vi "AlazarDSPSetParameterU32.vi"(4 "error in (no error)":errorcluster, 5 "value":u32, 6 "Parameter":u32(ring) items=["Raw+FFT supported", "FFT subtractor supported"], 7 "DSP Handle":u64) -> (0 "error out":errorcluster, 1 "Return Code":u32, 3 "DSP Handle":u64)   [LabVIEW 2009]
doc: "Get a device attribute as a signed long value."
uses:
  ATSApi.dll
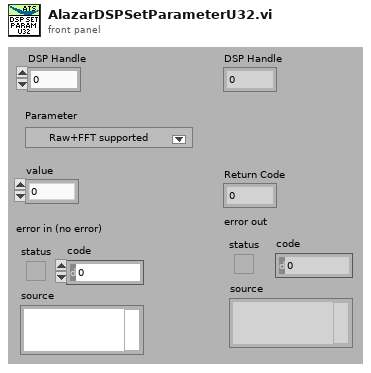
[diagram p1: front panel]
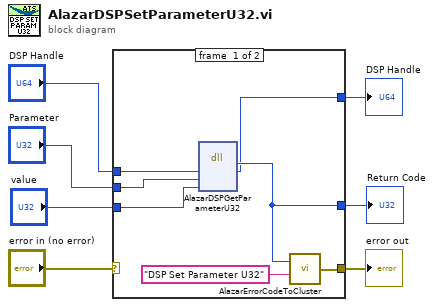
[diagram p0: block diagram]
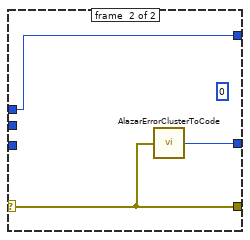
[diagram p2: hidden frame]
diagram:
  n1 = case shown="No Error" "error in (no error)" {
    selector: "error in (no error)" -> [_ w17]
    tunnel: [w11 w17] -> w6
    tunnel: [w13 w16] -> w5
    tunnel: "DSP Handle" -> [w14 w15]
    tunnel: [w10 w15] -> w3
    tunnel: "Parameter" -> [w9 _]
    tunnel: "value" -> [w8 _]
    frame #0 {
      n2 = dll-call lib="ATSApi.dll" fn="AlazarDSPGetParameterU32"("dspHandle"=w14, "parameter"=w9, "result"=w8) -> ("return type"=w13:u32, "dspHandle"=w10:u64)  [unwired: 5 in, 2 out]
      n3 = call "AlazarErrorCodeToCluster.vi"("Message"="DSP Set Parameter U32", "Error Code"=w13) -> ("error out"=w11:errorcluster)
    }
    frame #1 {
      (unwired) 0
      n4 = call "AlazarErrorClusterToCode.vi"("error in (no error)"=w17) -> ("Error Code"=w16:u32)
    }
  }
  "DSP Handle" <- w3
  "error out" <- w6
  "Return Code" <- w5
